vi "Run UTF Tests.vi"() -> ()   [LabVIEW 2014]
doc: "This VI will execute NI Unit Test Framework tests.\n\nArguments:\nLabVIEW project file path\nJUnit XML output file path"
uses:
  <vilib>/Wiresmith Technology/LabVIEW CLI/CLI Class/CLI.lvclass
  <vilib>/NI/UTF Junit Report/utf junit report.lvlib
panel:
  out "error out":errorcluster
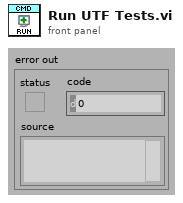
[diagram p1: front panel]
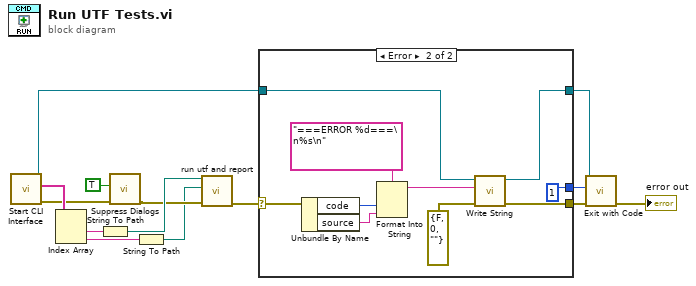
[diagram p0: block diagram]
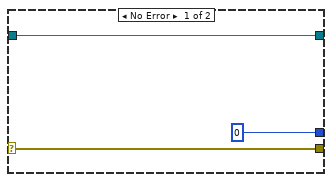
[diagram p2: hidden frame]
diagram:
  n1 = call <vilib>:"Start CLI Interface.vi"() -> ("error out"=w8:errorcluster, "Custom Parameters"=w13:string[], "CLI out"=w10:refnum<class "CLI.lvclass">)  [unwired: 9 in]
  n2 = Index Array(array=w13) -> (element #1=w14:string, element #2=w4:string)  [unwired: 2 in]
  n3 = String To Path(string=w14) -> (path=w6:path)
  n4 = call "Suppress Dialogs.vi"("error in (no error)"=w8, "Suppress Dialogs? (F)"=TRUE) -> ("error out"=w5:errorcluster)  [unwired: 9 in]
  n5 = String To Path(string=w4) -> (path=w3:path)
  n6 = call <vilib>:"run utf and report.vi"("error in (no error)"=w5, "junit report file path"=w3, "project file path"=w6) -> ("Error Out"=w2:errorcluster)  [unwired: 8 in]
  n7 = case shown="Error" w2 {
    selector: w2 -> [w17 w24]
    tunnel: w10 -> [w16 w20]
    tunnel: [w17 w23] -> w12
    tunnel: [w16 w22] -> w11
    tunnel: [0 1] -> w9
    frame No Error {
    }
    frame Error {
      n8 = Unbundle By Name(w24) -> ("code"=w25:i32, "source"=w27:string)
      n9 = Format Into String(format string="===ERROR %d===\n%s\n", w25, w27) -> (resulting string=w18:string)  [unwired: 2 in, 1 out]
      n10 = call <vilib>:"Write String.vi"("error in (no error)"=errorcluster {"status"=FALSE, "code"=0, "source"=""} ("error out"), "Text to Write"=w18, "CLI in"=w20) -> ("error out"=w23:errorcluster, "CLI out"=w22:refnum<class "CLI.lvclass">)  [unwired: 7 in]
    }
  }
  n11 = call <vilib>:"Exit with Code.vi"("error in (no error)"=w12, "Exit Code (0)"=w9, "CLI in"=w11) -> ("error out"=→"error out":errorcluster)  [unwired: 8 in]
